vi "Queue_Driver.vi"   [LabVIEW 2023]
doc: "Polymorphic VI to Use all the Queue Drivers"
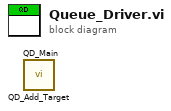
[diagram p0: block diagram]
diagram:
  n1 = call "QD_Add_Target.vi"() -> ()  [unwired: 13 in, 3 out]
  n2 = call "QD_Main.vi"() -> ()  [unwired: 13 in, 3 out]
